vi "Callback - Get Plottable Names.vi"(8 "error in (no error)":errorcluster, 11 "BluePlotHandleDemo in":refnum<class "NIringPlotHandle.lvclass">) -> (0 "error out":errorcluster, 2 "Plottable Names":string[](array[string]), 3 "BluePlotHandleDemo out":refnum<class "NIringPlotHandle.lvclass">)   [LabVIEW 2021, in "NIringPlotHandle.lvclass"]
uses:
  NIringPlotHandle.lvclass
  NIringPlotHandle.lvclass/NIringPlotHandle.ctl
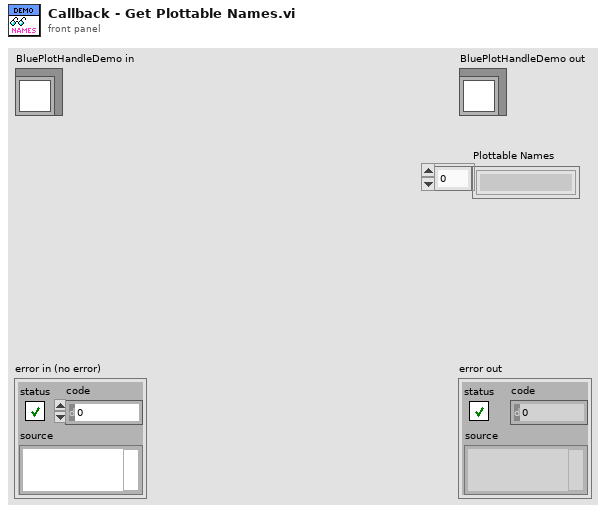
[diagram p1: front panel]
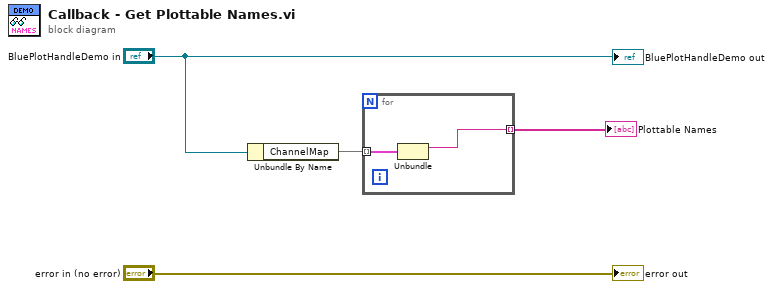
[diagram p0: block diagram]
diagram:
  n1 = Unbundle By Name("BluePlotHandleDemo in") -> ("ChannelMap"=w3:map{string, refnum<data-value>})
  n2 = for {
    tunnel: w3 -> [w6] mode=indexing
    tunnel: [w5] -> w2 mode=indexing
    n3 = Unbundle(w6) -> ("name"=w5:string)  [unwired: 1 out]
  }
  "Plottable Names" <- w2
  "error out" <- "error in (no error)"
  "BluePlotHandleDemo out" <- "BluePlotHandleDemo in"
